vi "1D Fit Unscale Fit Outputs v2.vi"(6 "# Points":i32, 7 "Fit Control Data in":T1, 8 "Error In":errorcluster, 9 "IRF Normalization Factor":dbl, 10 "Decay Normalization Factor":dbl, 11 "Fit Output in  (w sigma)":T5={"best nonlinear fit"=[], "best fit parameters"=[], "R^2"=0.0, "RMSE"=0.0, "error out"={"status"=FALSE, "code"=0, "source"=""}, "Fitting Method"=enum."Least Square", "number of function calls"=0, "number of iterations"=0, "covariance"=[], "Chi 2"=0.0, "DOF"=0, "Fit Convergence Criterion"=enum."Continue", "Fitting Algorithm"=enum."Levenberg-Marquardt", "Weighted Fit"=FALSE, "Gradient"=0.0, "|Delta Chi 2|"=0.0, "|Delta Chi 2|/Chi 2"=0.0, "Max |Delta a| /|a|"=0.0, "Lambda"=-1.0, "RSS"=0.0, "AIC"=0.0, "BIC"=0.0, "Max number of function calls"=0, "Max number of iterations"=0, "IRF"={"X Array"=[], "Y Array"=[]}, "IRF Normalization Factor"=0.0, "Decay Normalization Factor"=0.0}) -> (0 "Error Out":errorcluster, 1 "All unscaled parameters (w tau)":dbl[](array[numeric]), 2 "Fitted unscaled parameters (w tau)":dbl[](array[numeric]), 3 "Unscaled Fit Output out (w sigma)":T5={"best nonlinear fit"=[], "best fit parameters"=[], "R^2"=0.0, "RMSE"=0.0, "error out"={"status"=FALSE, "code"=0, "source"=""}, "Fitting Method"=enum."Least Square", "number of function calls"=0, "number of iterations"=0, "covariance"=[], "Chi 2"=0.0, "DOF"=0, "Fit Convergence Criterion"=enum."Continue", "Fitting Algorithm"=enum."Levenberg-Marquardt", "Weighted Fit"=FALSE, "Gradient"=0.0, "|Delta Chi 2|"=0.0, "|Delta Chi 2|/Chi 2"=0.0, "Max |Delta a| /|a|"=0.0, "Lambda"=-1.0, "RSS"=0.0, "AIC"=0.0, "BIC"=0.0, "Max number of function calls"=0, "Max number of iterations"=0, "IRF"={"X Array"=[], "Y Array"=[]}, "IRF Normalization Factor"=0.0, "Decay Normalization Factor"=0.0}, 5 "Fit Control Data out":T1)   [LabVIEW 2021, in "Fits.lvlib"]
uses:
  Fits.lvlib
  Non-linear Fit Output v3.ctl
  Nonlinear Fit Method.ctl
  <vilib>/Analysis/Matrix/Datatypes/RealMatrix.ctl
  Convergence Criteria.ctl
  Non-linear Fitting Algorithm.ctl
  Graphs/XY Graph/XY Plot Data.ctl
  Decay Convolution/Fit Control Data v2.ctl
  IRF(X)PSED/Decay Fit Parameters In List.ctl
  Decay Convolution/Decay Model.ctl
  <vilib>/Analysis/Matrix/NI_Matrix.lvlib
  Graphs/XY Graph/XY Graph Add-Ons.lvlib
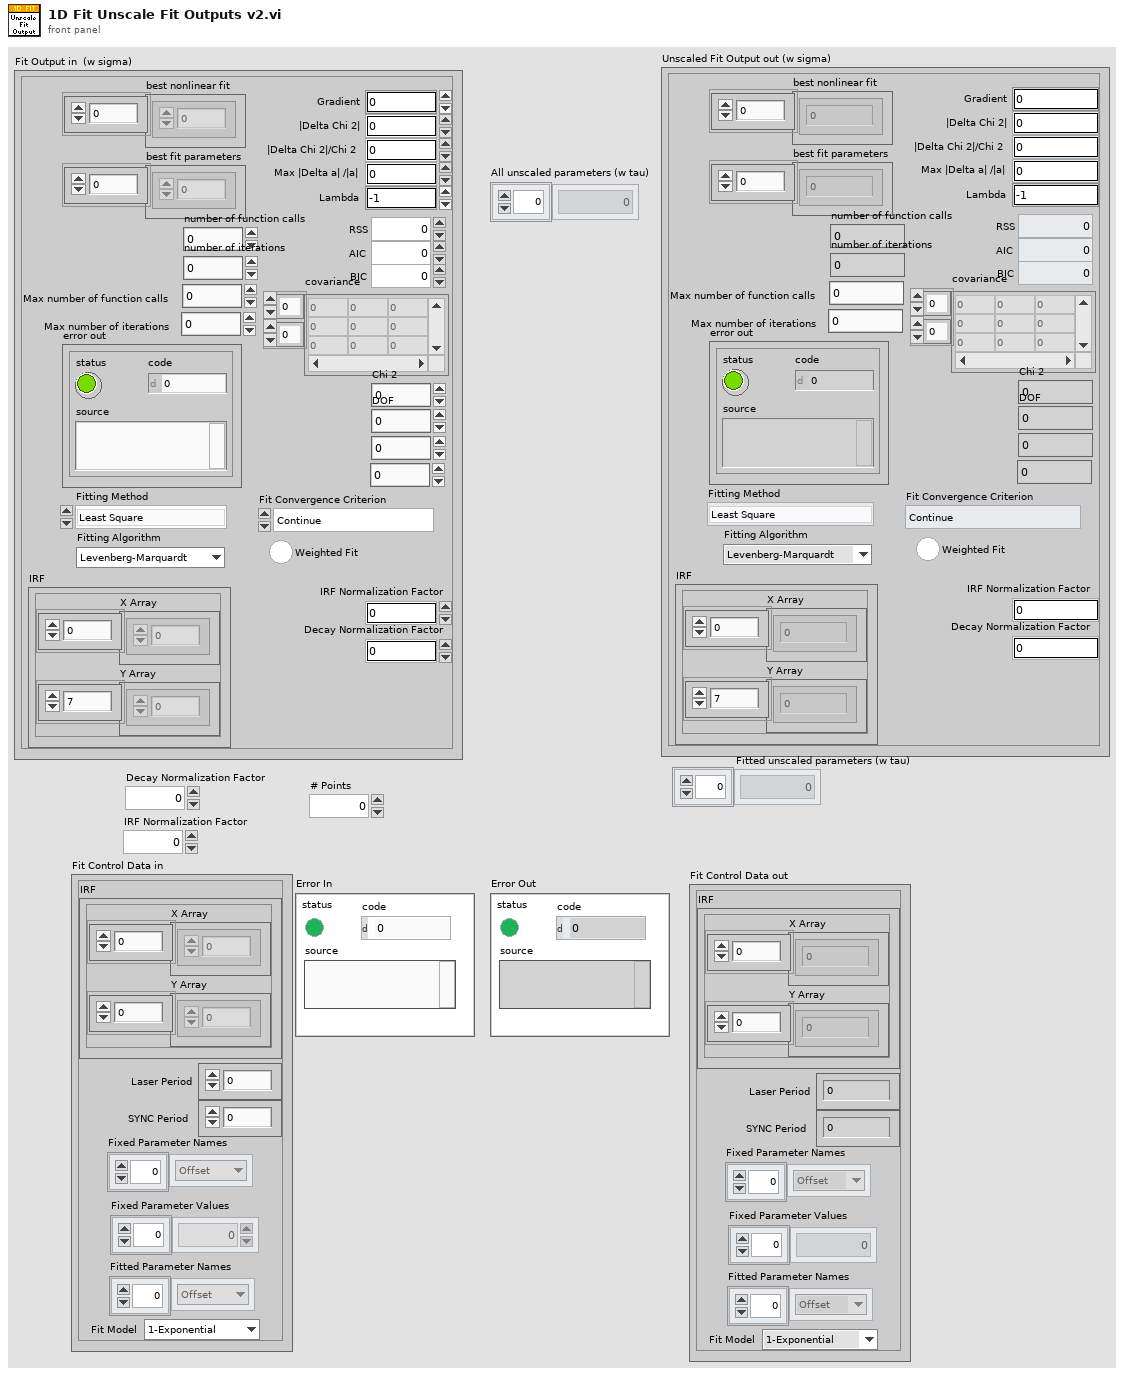
[diagram p1: front panel]
types:
  T1 = typedef "Fits.lvlib/Fit Control Data v2.ctl" = cluster{"IRF":T2, "Laser Period":dbl, "SYNC Period":dbl, "Fixed Parameter Names":T3[], "Fixed Parameter Values":dbl[], "Fitted Parameter Names":T3[], "Fit Model":T4}
  T2 = typedef "XY Graph Add-Ons.lvlib/XY Plot Data.ctl" = cluster{"X Array":dbl[], "Y Array":dbl[]}
  T3 = typedef "Fits.lvlib/Decay Fit Parameters In List.ctl" = enum16{"Offset", "Baseline", "A_1", "tau_1", "A_2", "tau_2"}
  T4 = typedef "Fits.lvlib/Decay Model.ctl" = enum16{"1-Exponential", "2-Exponentials"}
  T5 = typedef "Fits.lvlib/Non-linear Fit Output v3.ctl" = cluster{"best nonlinear fit":dbl[], "best fit parameters":dbl[], "R^2":dbl, "RMSE":dbl, "error out":errorcluster, "Fitting Method":T6, "number of function calls":i32, "number of iterations":i32, "covariance":T7, "Chi 2":dbl, "DOF":i32, "Fit Convergence Criterion":T8, "Fitting Algorithm":T9, "Weighted Fit":bool, "Gradient":dbl, "|Delta Chi 2|":dbl, "|Delta Chi 2|/Chi 2":dbl, "Max |Delta a| /|a|":dbl, "Lambda":dbl, "RSS":dbl, "AIC":dbl, "BIC":dbl, "Max number of function calls":i32, "Max number of iterations":i32, "IRF":T2, "IRF Normalization Factor":dbl, "Decay Normalization Factor":dbl}
  T6 = typedef "Fits.lvlib/Nonlinear Fit Method.ctl" = enum16{"Least Square", "Least Absolute Residual", "Bisquare", "MLE"}
  T7 = typedef "NI_Matrix.lvlib/RealMatrix.ctl" = dbl[][]
  T8 = typedef "Fits.lvlib/Convergence Criteria.ctl" = enum16{"Continue", "Tolerances Exceeded", "Max Time Exceeded", "Max Iterations Exceeded", "Max Function Evaluations Exceeded", "Scale Range Exceeded"}
  T9 = typedef "Fits.lvlib/Non-linear Fitting Algorithm.ctl" = enum16{"Levenberg-Marquardt", "Trust-Region Dogleg"}
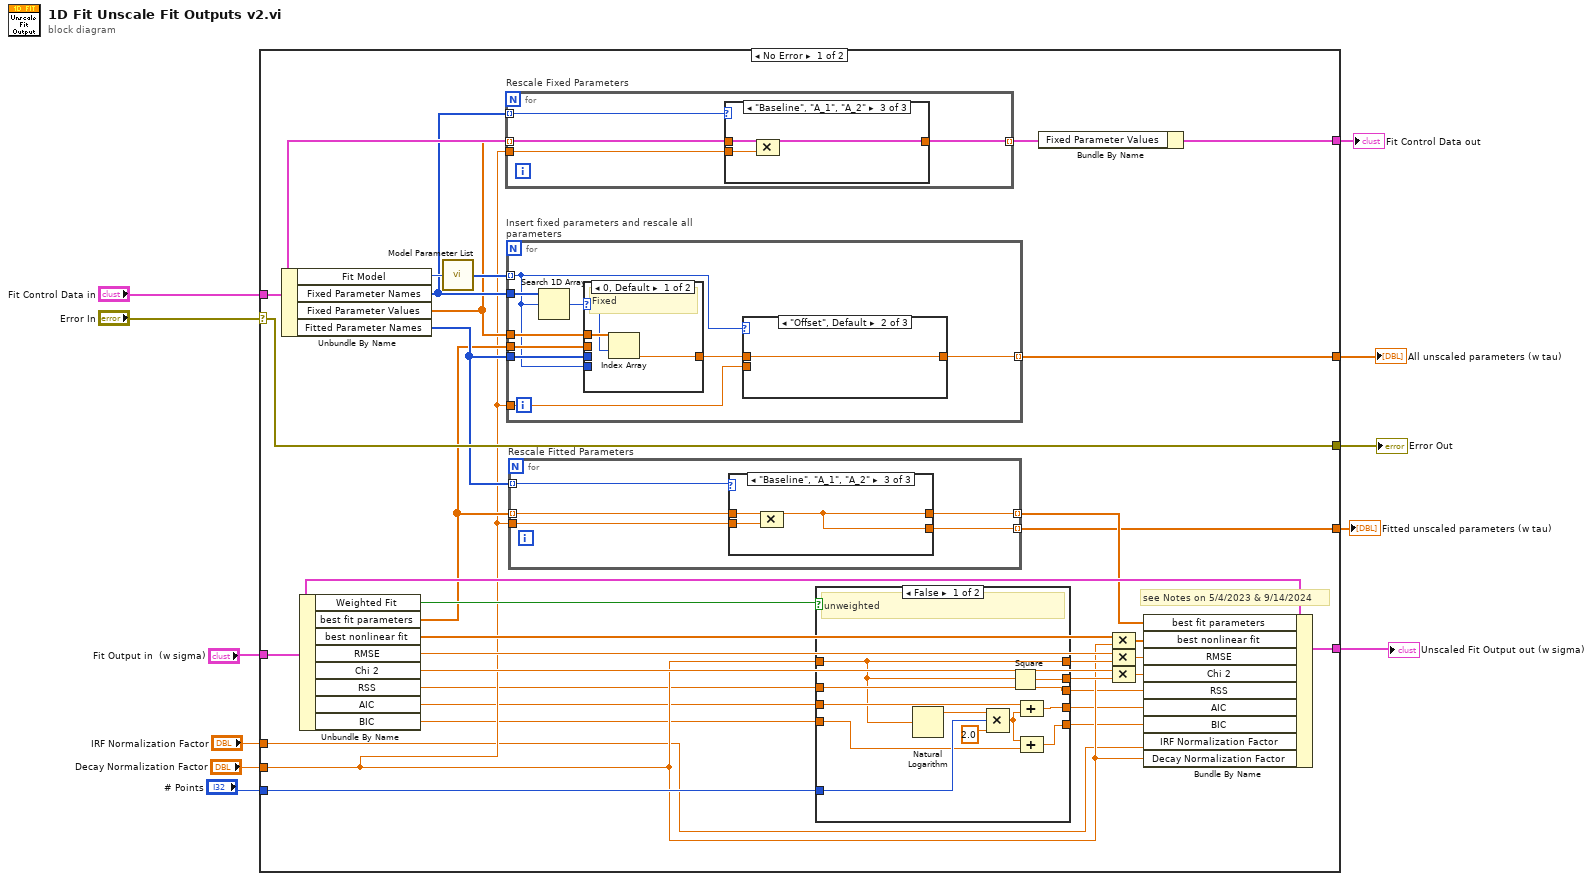
[diagram p0: block diagram]
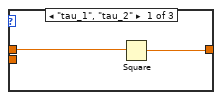
[diagram p2: hidden frame]
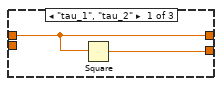
[diagram p4: hidden frame]
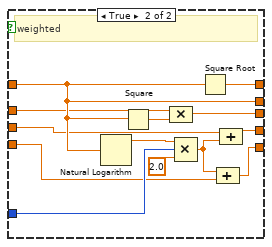
[diagram p6: hidden frame]
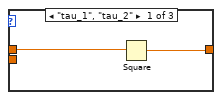
[diagram p7: hidden frame]
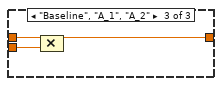
[diagram p8: hidden frame]
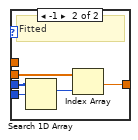
[diagram p9: hidden frame]
diagram:
  n1 = case shown="No Error" "Error In" {
    selector: "Error In" -> [w31 w114]
    tunnel: "Fit Output in  (w sigma)" -> [w44 _]
    tunnel: [w43 _] -> w10
    tunnel: "Fit Control Data in" -> [w26 w113]
    tunnel: [w30 _] -> w9
    tunnel: "IRF Normalization Factor" -> [w18 _]
    tunnel: "Decay Normalization Factor" -> [w19 _]
    tunnel: [w31 w114] -> w6
    tunnel: [w22 w113] -> w5
    tunnel: [w21 _] -> w2
    tunnel: "# Points" -> [w20 _]
    frame No Error {
      # "see Notes on 5/4/2023 & 9/14/2024"
      n2 = Unbundle By Name(w26) -> ("Fit Model"=w37:T4, "Fixed Parameter Names"=w25:T3[], "Fixed Parameter Values"=w24:dbl[], "Fitted Parameter Names"=w29:T3[])
      n3 = Unbundle By Name(w44) -> ("Weighted Fit"=w35:bool, "best fit parameters"=w28:dbl[], "best nonlinear fit"=w42:dbl[], "RMSE"=w40:dbl, "Chi 2"=w34:dbl, "RSS"=w17:dbl, "AIC"=w16:dbl, "BIC"=w15:dbl)
      n4 = call "Model Parameter List.vi"("Fit Model"=w37) -> ("Model Parameter List"=w38:T3[])
      n5 = for "Rescale Fixed Parameters" {
        tunnel: w25 -> [w48] mode=indexing
        tunnel: w24 -> [w47] mode=indexing
        tunnel: w19 -> [w46]
        tunnel: [w45] -> w23 mode=indexing
        n6 = case shown="\"Baseline\", \"A_1\", \"A_2\"" w48 {
          tunnel: w47 -> [w50 w51 w54]
          tunnel: w46 -> [_ _ w53]
          tunnel: [w49 w51 w52] -> w45
          frame "tau_1", "tau_2" {
            n7 = Square(x=w50) -> (x^2=w49:dbl)
          }
          frame "Offset", Default {
          }
          frame "Baseline", "A_1", "A_2" {
            n8 = Compound Arithmetic op=MULTIPLY(w54, w53) -> (w52:dbl)
          }
        }
      }
      n9 = for "Insert fixed parameters and rescale all parameters" {
        tunnel: w38 -> [w91] mode=indexing
        tunnel: w25 -> [w98]
        tunnel: w19 -> [w94]
        tunnel: w29 -> [w92]
        tunnel: w24 -> [w93]
        tunnel: w28 -> [w96]
        tunnel: [w90] -> w30 mode=indexing
        n10 = Search 1D Array(1D array=w98, element=w91) -> (index of element=w97:i32)  [unwired: 1 in]
        n11 = case shown="0, Default" w97 {
          selector: w97 -> [w106 _]
          tunnel: w96 -> [_ w110]
          tunnel: [w105 w108] -> w95
          tunnel: w93 -> [w107 _]
          tunnel: w92 -> [_ w112]
          tunnel: w91 -> [_ w111]
          frame 0, Default {
            # "Fixed"
            n12 = Index Array(array=w107, index=w106) -> (element=w105:dbl)
          }
          frame -1 {
            # "Fitted"
            n13 = Search 1D Array(1D array=w112, element=w111) -> (index of element=w109:i32)  [unwired: 1 in]
            n14 = Index Array(array=w110, index=w109) -> (element=w108:dbl)
          }
        }
        n15 = case shown="\"Offset\", Default" w91 {
          tunnel: w95 -> [w100 w101 w104]
          tunnel: w94 -> [_ _ w103]
          tunnel: [w99 w101 w102] -> w90
          frame "tau_1", "tau_2" {
            n16 = Square(x=w100) -> (x^2=w99:dbl)
          }
          frame "Offset", Default {
          }
          frame "Baseline", "A_1", "A_2" {
            n17 = Compound Arithmetic op=MULTIPLY(w104, w103) -> (w102:dbl)
          }
        }
      }
      n18 = for "Rescale Fitted Parameters" {
        tunnel: w29 -> [w59] mode=indexing
        tunnel: w28 -> [w58] mode=indexing
        tunnel: w19 -> [w57]
        tunnel: [w56] -> w27 mode=indexing
        tunnel: [w55] -> w21 mode=indexing
        n19 = case shown="\"Baseline\", \"A_1\", \"A_2\"" w59 {
          tunnel: w58 -> [w61 w62 w64]
          tunnel: w57 -> [_ _ w65]
          tunnel: [w61 w62 w63] -> w56
          tunnel: [w60 w62 w63] -> w55
          frame "tau_1", "tau_2" {
            n20 = Square(x=w61) -> (x^2=w60:dbl)
          }
          frame "Offset", Default {
          }
          frame "Baseline", "A_1", "A_2" {
            n21 = Compound Arithmetic op=MULTIPLY(w64, w65) -> (w63:dbl)
          }
        }
      }
      n22 = case shown="False" w35 {
        tunnel: w19 -> [w70 w84]
        tunnel: [w70 w89] -> w36
        tunnel: [w76 w84] -> w32
        tunnel: w20 -> [w68 w83]
        tunnel: w17 -> [w72 w81]
        tunnel: w16 -> [w71 w80]
        tunnel: w15 -> [w67 w78]
        tunnel: [w72 w82] -> w14
        tunnel: [w69 w79] -> w13
        tunnel: [w66 w77] -> w12
        frame False {
          # "unweighted"
          n23 = Natural Logarithm(1:w70) -> (0:w75:dbl)
          n24 = Compound Arithmetic op=MULTIPLY(w75, w68, 2.0 ("value")) -> (w73:dbl)
          n25 = Square(x=w70) -> (x^2=w76:dbl)
          n26 = Compound Arithmetic op=ADD(w71, w73) -> (w69:dbl)
          n27 = Compound Arithmetic op=ADD(w73, w67) -> (w66:dbl)
        }
        frame True {
          # "weighted"
          n28 = Natural Logarithm(1:w84) -> (0:w87:dbl)
          n29 = Square(x=w84) -> (x^2=w88:dbl)
          n30 = Compound Arithmetic op=MULTIPLY(w81, w88) -> (w82:dbl)
          n31 = Compound Arithmetic op=MULTIPLY(w87, w83, 2.0 ("value")) -> (w85:dbl)
          n32 = Square Root(x=w84) -> (sqrt(x)=w89:dbl)
          n33 = Compound Arithmetic op=ADD(w85, w78) -> (w77:dbl)
          n34 = Compound Arithmetic op=ADD(w80, w85) -> (w79:dbl)
        }
      }
      n35 = Bundle By Name(cluster=w26, "Fixed Parameter Values"=w23) -> (w22:T1)
      n36 = Compound Arithmetic op=MULTIPLY(w42, w19) -> (w41:dbl[])
      n37 = Compound Arithmetic op=MULTIPLY(w40, w36) -> (w39:dbl)
      n38 = Compound Arithmetic op=MULTIPLY(w34, w32) -> (w33:dbl)
      n39 = Bundle By Name(cluster=w44, "best fit parameters"=w27, "best nonlinear fit"=w41, "RMSE"=w39, "Chi 2"=w33, "RSS"=w14, "AIC"=w13, "BIC"=w12, "IRF Normalization Factor"=w18, "Decay Normalization Factor"=w19) -> (w43:T5)
    }
    frame Error {
    }
  }
  "Unscaled Fit Output out (w sigma)" <- w10
  "All unscaled parameters (w tau)" <- w9
  "Error Out" <- w6
  "Fit Control Data out" <- w5
  "Fitted unscaled parameters (w tau)" <- w2
